vi "normalize_vector.vi"(10 "Vector":cluster{"X":sgl, "Y":sgl, "Z":sgl}) -> (2 "Normalized Vector":cluster{"X":sgl, "Y":sgl, "Z":sgl})   [LabVIEW 2020, in "3DPC_SurfacePlot.xctl"]
uses:
  <vilib>/Native 3D Graph/xcontrol/3DPC_SurfacePlot.xctl
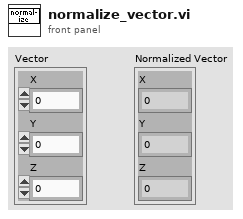
[diagram p1: front panel]
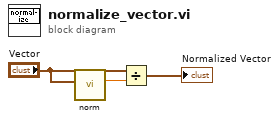
[diagram p0: block diagram]
diagram:
  n1 = call <vilib>:"norm.vi"("Vector"="Vector") -> ("Norm"=w1:sgl)  [unwired: 10 out]
  n2 = Divide(x="Vector", y=w1) -> (x/y=→"Normalized Vector":cluster{"X":sgl, "Y":sgl, "Z":sgl})
